vi "set to channel A.vi"(8 "error in (no error)":errorcluster) -> (0 "error out":errorcluster)   [LabVIEW 2010]
panel:
  out "Channel C":bool
  out "Channel B":bool
  out "Channel A":bool
  out "result array":string[](array[string])
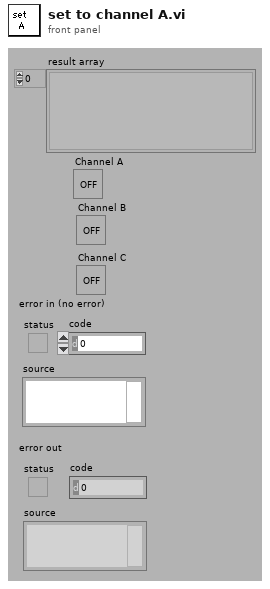
[diagram p1: front panel]
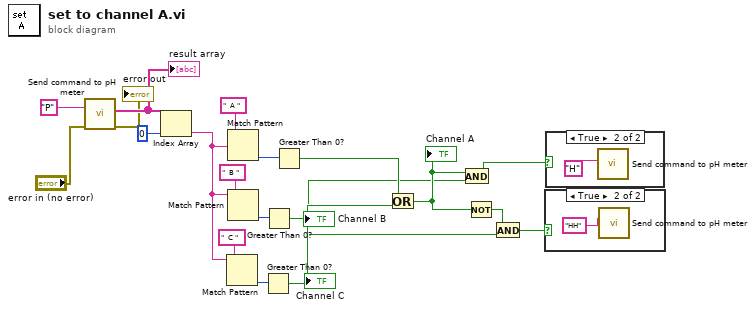
[diagram p0: block diagram]
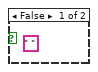
[diagram p2: hidden frame]
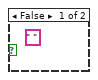
[diagram p3: hidden frame]
diagram:
  n1 = call "Send command to pH meter"("error in (no error)"="error in (no error)", "string to write"="P") -> ("error out"=→"error out":errorcluster, "result array"=w18:string[])  [unwired: 8 in]
  "result array" <- w18
  n2 = Index Array(array=w18, index=0) -> (element=w9:string)
  n3 = Match Pattern(string=w9, regular expression="  C ") -> (offset past match=w11:i32)  [unwired: 1 in, 3 out]
  n4 = Match Pattern(string=w9, regular expression="  A ") -> (offset past match=w14:i32)  [unwired: 1 in, 3 out]
  n5 = Match Pattern(string=w9, regular expression="  B ") -> (offset past match=w13:i32)  [unwired: 1 in, 3 out]
  n6 = Greater Than 0?(x=w11) -> (x > 0?=w12:bool)
  "Channel C" <- w12
  n7 = Greater Than 0?(x=w13) -> (x > 0?=w5:bool)
  "Channel B" <- w5
  n8 = Greater Than 0?(x=w14) -> (x > 0?=w8:bool)
  n9 = Or(x=w8, y=w12) -> (x .or. y?=w6:bool)
  "Channel A" <- w6
  n10 = And(x=w6, y=w5) -> (x .and. y?=w7:bool)
  n11 = Not(x=w6) -> (.not. x?=w4:bool)
  n12 = And(x=w4, y=w5) -> (x .and. y?=w3:bool)
  n13 = case shown="True" w3 {
    frame False {
      (unwired) " "
    }
    frame True {
      n14 = call "Send command to pH meter"("string to write"="HH") -> ()  [unwired: 9 in, 2 out]
    }
  }
  n15 = case shown="True" w7 {
    frame False {
      (unwired) " "
    }
    frame True {
      n16 = call "Send command to pH meter"("string to write"="H") -> ()  [unwired: 9 in, 2 out]
    }
  }
